vi "Get Title.vi"(11 "Bark in":refnum<class "Bark.lvclass">) -> (2 "Title":string, 3 "Bark out":refnum<class "Bark.lvclass">)   [LabVIEW 2016, in "Bark.lvlib" / "Bark.lvclass"]
uses:
  Bark.lvclass
  Bark.lvclass/Bark.ctl
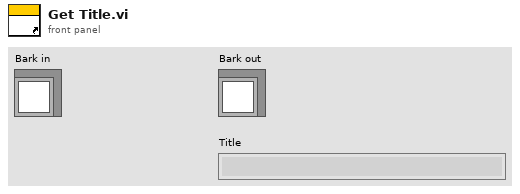
[diagram p1: front panel]
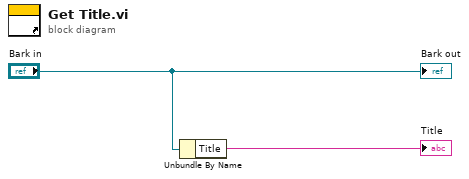
[diagram p0: block diagram]
diagram:
  n1 = Unbundle By Name("Bark in") -> ("Title"=→"Title":string)
  "Bark out" <- "Bark in"
